vi "FlatToRichni_xnet_can_bm_api_CanCommState.vi"(5 "OutputClusterType":T1, 11 "InputCluster":T4) -> (3 "OutputCluster":T1)   [LabVIEW 2025, in "xnet_can_bus_monitor_api_client.lvlib"]
uses:
  xnet_can_bus_monitor_api_client.lvlib
  ni_xnet_can_bm_api_CanCommState_Flat.ctl
  ni_xnet_can_bm_api_CommState.ctl
  ni_xnet_can_bm_api_LastCommError.ctl
  ni_xnet_can_bm_api_CanCommState.ctl
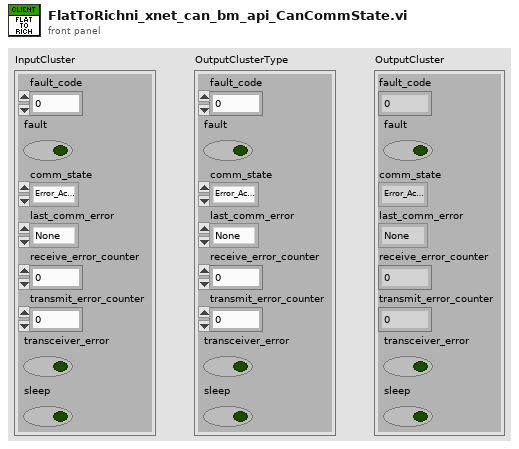
[diagram p1: front panel]
types:
  T1 = typedef "xnet_can_bus_monitor_api_client.lvlib/ni_xnet_can_bm_api_CanCommState.ctl" = cluster{"fault_code":i32, "fault":bool, "comm_state":T2, "last_comm_error":T3, "receive_error_counter":u32, "transmit_error_counter":u32, "transceiver_error":bool, "sleep":bool}
  T2 = typedef "xnet_can_bus_monitor_api_client.lvlib/ni_xnet_can_bm_api_CommState.ctl" = enum32{"Error_Active", "Error_Passive", "Bus_Off", "Init"}
  T3 = typedef "xnet_can_bus_monitor_api_client.lvlib/ni_xnet_can_bm_api_LastCommError.ctl" = enum32{"None", "Stuff", "Form", "ACK", "Bit1", "Bit0", "CRC"}
  T4 = typedef "xnet_can_bus_monitor_api_client.lvlib/ni_xnet_can_bm_api_CanCommState_Flat.ctl" = cluster{"fault_code":i32, "fault":bool, "comm_state":T2, "last_comm_error":T3, "receive_error_counter":u32, "transmit_error_counter":u32, "transceiver_error":bool, "sleep":bool}
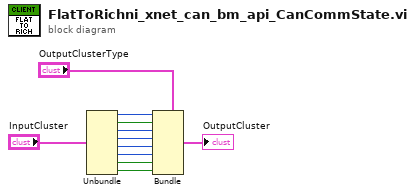
[diagram p0: block diagram]
diagram:
  n1 = Unbundle "Unbundle"("InputCluster") -> ("fault_code"=w8:i32, "fault"=w7:bool, "comm_state"=w6:T2, "last_comm_error"=w5:T3, "receive_error_counter"=w4:u32, "transmit_error_counter"=w3:u32, "transceiver_error"=w2:bool, "sleep"=w1:bool)
  n2 = Bundle "Bundle"(cluster="OutputClusterType", "fault_code"=w8, "fault"=w7, "comm_state"=w6, "last_comm_error"=w5, "receive_error_counter"=w4, "transmit_error_counter"=w3, "transceiver_error"=w2, "sleep"=w1) -> (→"OutputCluster":T1)
